vi "Result_Test.vi"(8 "error in (no error)":errorcluster caption="entrée d'erreur (pas d'erreur)", 11 "Get_Voltage en entrée":refnum<class "Read_Weight.lvclass">) -> (0 "error out":errorcluster caption="sortie d'erreur", 3 "Get_Voltage en sortie":refnum<class "Read_Weight.lvclass">)   [LabVIEW 2020, in "Library Test.lvlib" / "Read_Weight.lvclass"]
uses:
  Read_Weight.lvclass
  C:/Users/ngarcin/OneDrive - Altyor/Standard TB/Suite TB45/Class/Test/Test (Default)/Test (Default).lvclass
  Commun VI/TypeDef/Variable Printable.ctl
  Test_Wtih_Instr/Test_With_Inst.lvclass
  Commun VI/Library Commun.lvlib
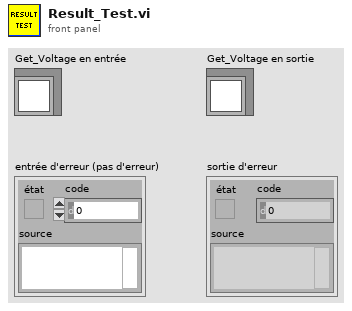
[diagram p1: front panel]
types:
  T1 = typedef "Variable Printable.ctl" = string
  T2 = enum16{"Get Variable", "Get All Variables", "Set Variable", "Delete Variable", "Delete All Variable"}
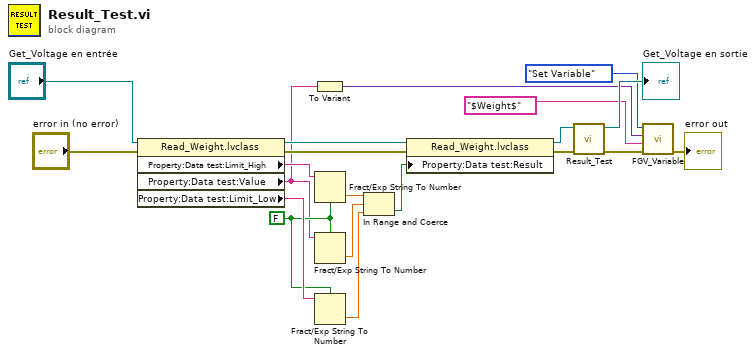
[diagram p0: block diagram]
diagram:
  w7 = FALSE ("utiliser le séparateur décimal du système (V)")
  n1 = property class="Read_Weight.lvclass"(reference="Get_Voltage en entrée", error in="error in (no error)") -> (reference out=w15:refnum<class "Read_Weight.lvclass">, error out=w13:errorcluster, "Property:Data test:Limit_High"=w20:string, "Property:Data test:Value"=w4:string, "Property:Data test:Limit_Low"=w19:string)
  n2 = To Variant(anything=w4) -> (Variant=w5:variant)
  n3 = Fract/Exp String To Number(use system decimal point (T)=w7, string=w20) -> (number=w18:dbl)  [unwired: 2 in, 1 out]
  n4 = Fract/Exp String To Number(use system decimal point (T)=w7, string=w4) -> (number=w17:dbl)  [unwired: 2 in, 1 out]
  n5 = Fract/Exp String To Number(use system decimal point (T)=w7, string=w19) -> (number=w16:dbl)  [unwired: 2 in, 1 out]
  n6 = In Range and Coerce(upper limit=w18, x=w17, lower limit=w16) -> (In Range?=w14:bool)  [unwired: 1 out]
  n7 = property class="Read_Weight.lvclass"(reference=w15, error in=w13, "Property:Data test:Result"=w14) -> (reference out=w8:refnum<class "Read_Weight.lvclass">, error out=w10:errorcluster)
  n8 = call-parent "Result_Test.vi"("error in (no error)"=w10, "Test_With_Inst en entrée"=w8) -> ("error out"=w3:errorcluster, "Test_With_Inst en sortie"=→"Get_Voltage en sortie":refnum<class "Read_Weight.lvclass">)  [unwired: 8 in]
  n9 = call "FGV_Variable.vi"("error in (no error)"=w3, "Variable"=T1 "$Weight$", "Data In"=w5, "Function"=T2."Set Variable") -> ("error out"=→"error out":errorcluster)  [unwired: 5 in, 2 out]
